vi "Read EQ data.vi"(8 "error in (no error)":errorcluster, 11 "file path":path) -> (0 "error out":errorcluster, 1 "gain correction (x/y)":dbl[](array[numeric]), 2 "frequency":dbl[](array[numeric]))   [LabVIEW 2022 SP3]
uses:
  <vilib>/Utility/file.llb/Read Delimited Spreadsheet (DBL).vi
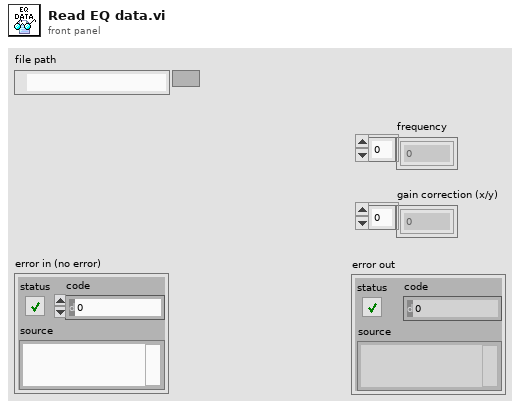
[diagram p1: front panel]
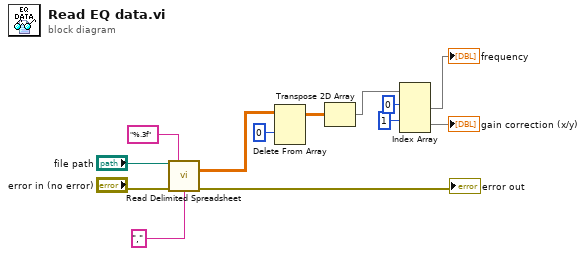
[diagram p0: block diagram]
diagram:
  n1 = call-poly <vilib>:"Read Delimited Spreadsheet.vi"("file path (dialog if empty)"="file path", "format (%.3f)"="%.3f", "error in (no error)"="error in (no error)", "delimiter (\\t)"="," ("delimiter (\\t)")) -> ("all rows"=w8:dbl[][], "error out"=→"error out":errorcluster)  [unwired: 6 in, 4 out]
  n2 = Delete From Array(array=w8, index (row)=0) -> (array with subset deleted=w6:dbl[][])  [unwired: 2 in, 1 out]
  n3 = Transpose 2D Array(2D array=w6) -> (transposed array=w5:dbl[][])
  n4 = Index Array(array=w5, index (row) #1=0 ("index (row)"), index (row) #2=1 ("index (row)")) -> (element #1=→"frequency":dbl[], element #2=→"gain correction (x/y)":dbl[])  [unwired: 2 in]
